vi "3.labtask3 (1).vi"() -> ()   [LabVIEW 2022 SP3]
uses:
  <vilib>/Utility/file.llb/Write Delimited Spreadsheet (DBL).vi
panel:
  out "Scalar":dbl
  in  "file path (dialog if empty)":path
  out "Array":dbl[](array[numeric])
  out "Waveform Chart":dynamicdata(graph)
  out "Total execution time (s)":u32
  out "Sampling period (ms)":dbl
  out "Total number of samples":dbl
  in  "Sampling rate (Hz)":dbl
  in  "Total duration (s)":dbl
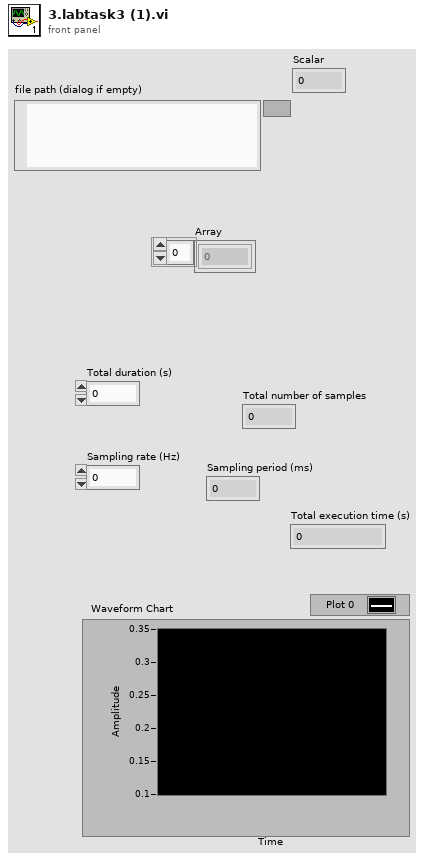
[diagram p1: front panel]
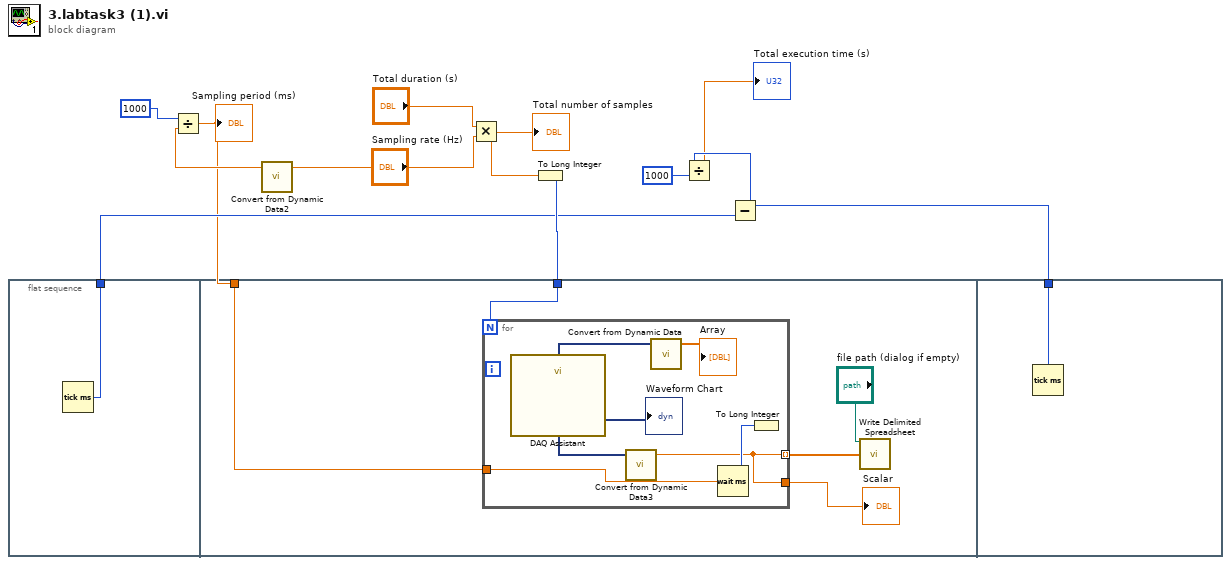
[diagram p0: block diagram]
diagram:
  n1 = flat-sequence {
    tunnel: [w12] -> w2
    tunnel: w7 -> [w17]
    tunnel: w1 -> [w16]
    tunnel: [w23] -> w3
    frame #0 {
      n2 = Tick Count (ms)() -> (millisecond timer value=w12:u32)
    }
    frame #1 {
      n3 = for {
        N: w17 -> [_]
        tunnel: w16 -> [w22]
        tunnel: [w18] -> w14 mode=indexing
        tunnel: [w18] -> w13
        n4 = call "DAQ Assistant"() -> ("data"=w19:dynamicdata)  [unwired: 17 in, 2 out]
        "Waveform Chart" <- w19
        n5 = call "Convert from Dynamic Data3"("Dynamic Data Type"=w19) -> ("Scalar"=w18:dbl)  [unwired: 3 in]
        n6 = call "Convert from Dynamic Data"("Dynamic Data Type"=w19) -> ("Array"=→"Array":dbl[])  [unwired: 3 in]
        n7 = Wait (ms)(milliseconds to wait=w22) -> (millisecond timer value=w21:u32)
        n8 = To Long Integer(number=w21) -> ()  [unwired: 1 out]
      }
      "Scalar" <- w13
      n9 = call-poly <vilib>:"Write Delimited Spreadsheet.vi"("file path (dialog if empty)"="file path (dialog if empty)", "1D data"=w14) -> ()  [unwired: 12 in, 2 out]
    }
    frame #2 {
      n10 = Tick Count (ms)() -> (millisecond timer value=w23:u32)
    }
  }
  n11 = Divide(x=1000, y="Sampling rate (Hz)") -> (x/y=w1:dbl)
  "Sampling period (ms)" <- w1
  n12 = call "Convert from Dynamic Data2"() -> ()  [unwired: 4 in, 1 out]
  n13 = Multiply(x="Total duration (s)", y="Sampling rate (Hz)") -> (x*y=w11:dbl)
  "Total number of samples" <- w11
  n14 = To Long Integer(number=w11) -> (32bit integer=w7:i32)
  n15 = Subtract(x=w3, y=w2) -> (x-y=w6:u32)
  n16 = Divide(x=w6, y=u32 1000) -> (x/y=→"Total execution time (s)":dbl)
